vi "Write trigger level  (0.0 V).vi"(8 "error in (no error)":errorcluster, 10 "trigger level  (0.0 V)":dbl[unit] format="%.3f", 11 "Configure Edge Trigger Source Msg in":refnum<class "Configure Edge Trigger Source Msg.lvclass">) -> (0 "error out":errorcluster, 3 "Configure Edge Trigger Source Msg out":refnum<class "Configure Edge Trigger Source Msg.lvclass">)   [LabVIEW 2014, in "CS++Scope.lvlib" / "Configure Edge Trigger Source Msg.lvclass"]
uses:
  Configure Edge Trigger Source Msg.lvclass
  Configure Edge Trigger Source Msg.lvclass/Configure Edge Trigger Source Msg.ctl
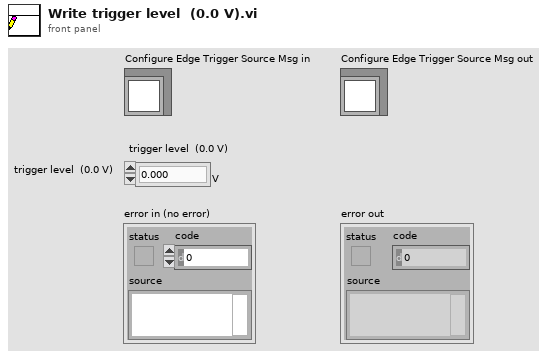
[diagram p1: front panel]
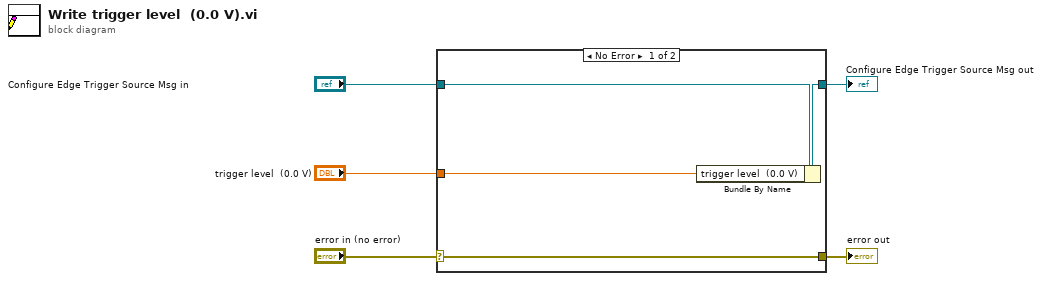
[diagram p0: block diagram]
diagram:
  n1 = case shown="No Error" "error in (no error)" {
    selector: "error in (no error)" -> [w9 w10]
    tunnel: [w9 w10] -> w4
    tunnel: [w7 w11] -> w2
    tunnel: "Configure Edge Trigger Source Msg in" -> [w8 w11]
    tunnel: "trigger level  (0.0 V)" -> [w6 _]
    frame No Error {
      n2 = Bundle By Name(cluster=w8, "trigger level  (0.0 V)"=w6) -> (w7:refnum<class "Configure Edge Trigger Source Msg.lvclass">)
    }
    frame Error {
    }
  }
  "error out" <- w4
  "Configure Edge Trigger Source Msg out" <- w2
